vi "sortGetConfig.vi"(11 "config data in":T1={"filterWheels"=[], "gratings"=[{"blaze"=0, "grooveDensity"=1800, "positionIndex"=0}, {"blaze"=0, "grooveDensity"=1200, "positionIndex"=1}, {"blaze"=0, "grooveDensity"=300, "positionIndex"=2}], "mirrors"=[{"locationId"=1}, {"locationId"=2}], "model"="iHR320", "ports"=[{"locationId"=1, "slitType"=2}, {"locationId"=2, "slitType"=2}, {"locationId"=4, "slitType"=2}], "productId"="", "serialNumber"=""}) -> (3 "config data out":T1)   [LabVIEW 2023, in "Monochromator.lvclass"]
uses:
  Monochromator.lvclass
  Monochromator.lvclass/Monochromator.ctl
  filterWheel.ctl
  grating.ctl
  mirror.ctl
  port.ctl
  configuration.ctl
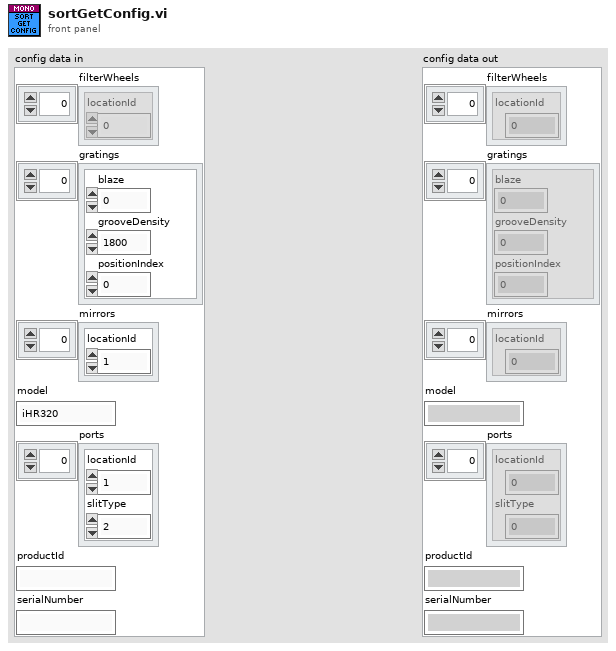
[diagram p1: front panel]
types:
  T1 = typedef "Monochromator.lvclass/configuration.ctl" = cluster{"filterWheels":T2[], "gratings":T3[], "mirrors":T4[], "model":string, "ports":T5[], "productId":string, "serialNumber":string}
  T2 = typedef "Monochromator.lvclass/filterWheel.ctl" = cluster{"locationId":i32}
  T3 = typedef "Monochromator.lvclass/grating.ctl" = cluster{"blaze":i32, "grooveDensity":i32, "positionIndex":i32}
  T4 = typedef "Monochromator.lvclass/mirror.ctl" = cluster{"locationId":i32}
  T5 = typedef "Monochromator.lvclass/port.ctl" = cluster{"locationId":i32, "slitType":i32}
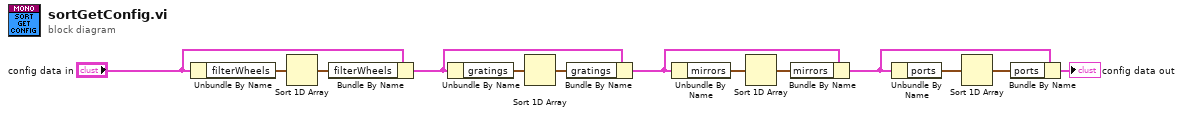
[diagram p0: block diagram]
diagram:
  n1 = Unbundle By Name("config data in") -> ("filterWheels"=w13:T2[])
  n2 = Sort 1D Array(array=w13) -> (sorted array=w12:T2[])
  n3 = Bundle By Name(cluster="config data in", "filterWheels"=w12) -> (w8:T1)
  n4 = Unbundle By Name(w8) -> ("gratings"=w10:T3[])
  n5 = Sort 1D Array(array=w10) -> (sorted array=w9:T3[])
  n6 = Bundle By Name(cluster=w8, "gratings"=w9) -> (w5:T1)
  n7 = Unbundle By Name(w5) -> ("mirrors"=w6:T4[])
  n8 = Sort 1D Array(array=w6) -> (sorted array=w7:T4[])
  n9 = Bundle By Name(cluster=w5, "mirrors"=w7) -> (w2:T1)
  n10 = Unbundle By Name(w2) -> ("ports"=w4:T5[])
  n11 = Sort 1D Array(array=w4) -> (sorted array=w3:T5[])
  n12 = Bundle By Name(cluster=w2, "ports"=w3) -> (→"config data out":T1)
